vi "Sel UnSel Switch.vi"(8 "error in (no error)":errorcluster, 10 "Point":T1, 11 "Methods ListCtrl":refnum<vi>) -> (0 "error out":errorcluster, 3 "Methods ListCtrl 2":refnum<vi>)   [LabVIEW 2020, in "WebServiceImporter.lvlib" / "Main Panel.lvlib" / "Select Methods.lvlib"]
uses:
  <vilib>/Platform/WebService/Main Panel/Pages/Select Methods/Select Methods.lvlib
  <vilib>/Utility/miscctls.llb/LVPositionTypeDef.ctl
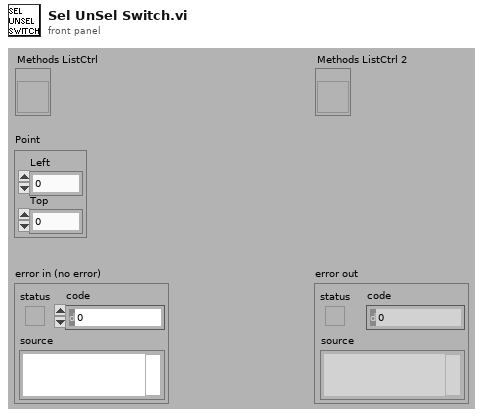
[diagram p1: front panel]
types:
  T1 = typedef "LVPositionTypeDef.ctl" = cluster{"Left":i32, "Top":i32}
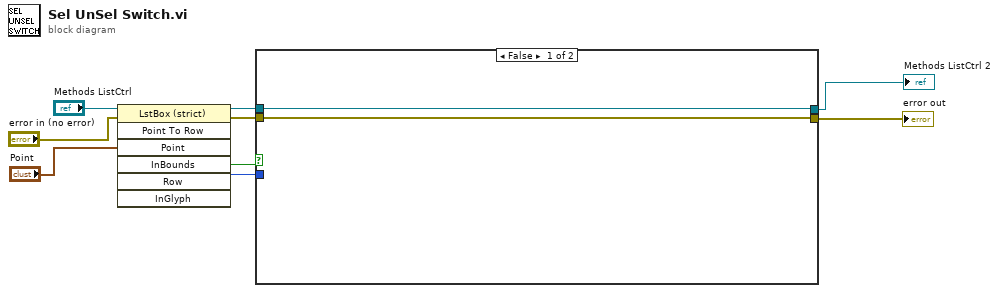
[diagram p0: block diagram]
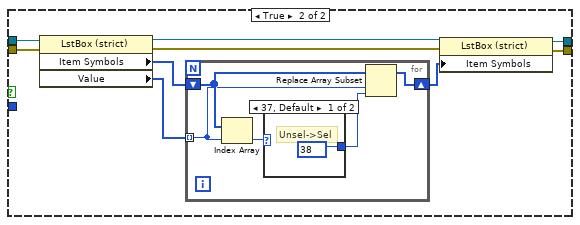
[diagram p2: hidden frame]
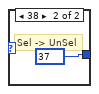
[diagram p3: hidden frame]
diagram:
  n1 = invoke class="LstBox (strict)" method="Point To Row"(reference="Methods ListCtrl", error in="error in (no error)", "Point"="Point") -> (reference out=w5:refnum<vi>, error out=w4:errorcluster, "InBounds"=w6:bool, "Row"=w3:i32)  [unwired: 4 in, 3 out]
  n2 = case shown="False" w6 {
    tunnel: w5 -> [w11 w20]
    tunnel: w4 -> [w10 w19]
    tunnel: w3 -> [_ _]
    tunnel: [w11 w13] -> w1
    tunnel: [w10 w12] -> w2
    frame False {
    }
    frame True {
      n3 = property class="LstBox (strict)"(reference=w20, error in=w19) -> (reference out=w16:refnum<vi>, error out=w15:errorcluster, "Item Symbols"=w17:i32[], "Value"=w18:i32[])
      n4 = for {
        tunnel: w18 -> [w23] mode=indexing
        shift-right: [w21] -> w14
        shift-left: w17 -> [w24]
        n5 = Index Array(array=w24, index=w23) -> (element=w25:i32)
        n6 = case shown="37, Default" w25 {
          tunnel: [38 37] -> w22
          frame 37, Default {
            # "Unsel->Sel"
          }
          frame 38 {
            # "Sel -> UnSel"
          }
        }
        n7 = Replace Array Subset(array=w24, new element=w22, index=w23) -> (w21:i32[])
      }
      n8 = property class="LstBox (strict)"(reference=w16, error in=w15, "Item Symbols"=w14) -> (reference out=w13:refnum<vi>, error out=w12:errorcluster)
    }
  }
  "error out" <- w2
  "Methods ListCtrl 2" <- w1
